vi "feux_rouge.vi"() -> ()   [LabVIEW 2018]
uses:
  F_r_var_glob.vi
panel:
  in  "stop":bool
  in  "Boolean 3":bool
  in  "Boolean 2":bool
  in  "Boolean":bool
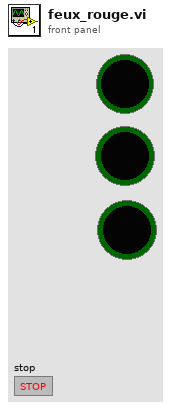
[diagram p1: front panel]
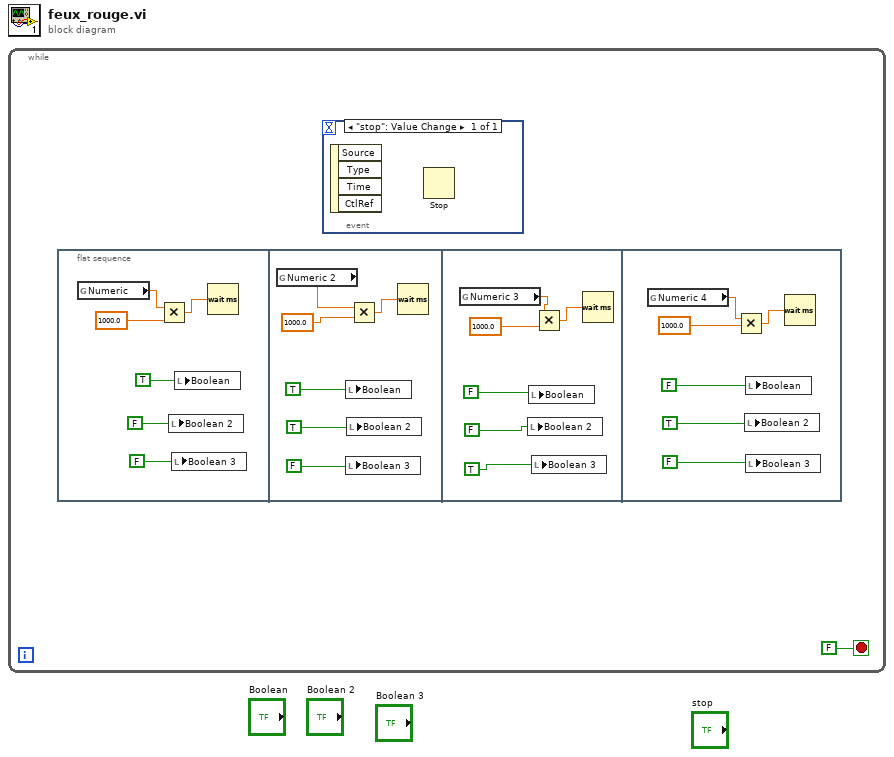
[diagram p0: block diagram]
diagram:
  n1 = while {
    stop <- FALSE stop-if-true
    n2 = flat-sequence {
      frame #0 {
        n3 = global read "F_r_var_glob.vi" "Numeric"() -> (w7:dbl)
        n4 = Multiply(x=w7, y=1000.0) -> (x*y=w5:dbl)
        n5 = local write "Boolean 2"(FALSE) -> ()
        n6 = local write "Boolean 3"(FALSE) -> ()
        n7 = local write "Boolean"(TRUE) -> ()
        n8 = Wait (ms)(milliseconds to wait=w5) -> ()  [unwired: 1 out]
      }
      frame #1 {
        n9 = global read "F_r_var_glob.vi" "Numeric 2"() -> (w11:dbl)
        n10 = local write "Boolean"(TRUE) -> ()
        n11 = local write "Boolean 3"(FALSE) -> ()
        n12 = local write "Boolean 2"(TRUE) -> ()
        n13 = Multiply(x=w11, y=1000.0) -> (x*y=w13:dbl)
        n14 = Wait (ms)(milliseconds to wait=w13) -> ()  [unwired: 1 out]
      }
      frame #2 {
        n15 = global read "F_r_var_glob.vi" "Numeric 3"() -> (w14:dbl)
        n16 = local write "Boolean 2"(FALSE) -> ()
        n17 = local write "Boolean"(FALSE) -> ()
        n18 = local write "Boolean 3"(TRUE) -> ()
        n19 = Multiply(x=w14, y=1000.0) -> (x*y=w16:dbl)
        n20 = Wait (ms)(milliseconds to wait=w16) -> ()  [unwired: 1 out]
      }
      frame #3 {
        n21 = global read "F_r_var_glob.vi" "Numeric 4"() -> (w21:dbl)
        n22 = Multiply(x=w21, y=1000.0) -> (x*y=w22:dbl)
        n23 = local write "Boolean 2"(TRUE) -> ()
        n24 = local write "Boolean"(FALSE) -> ()
        n25 = local write "Boolean 3"(FALSE) -> ()
        n26 = Wait (ms)(milliseconds to wait=w22) -> ()  [unwired: 1 out]
      }
    }
    n27 = event shown="[0] \"stop\": Value Change" {
      selector: _ -> [_]
      dyn-events: _ -> [_]
      timeout: _ -> [_]
      event "stop": Value Change {
        n28 = event-data() -> ()  [unwired: 1 in, 4 out]
        n29 = Stop() -> ()  [unwired: 1 in]
      }
    }
  }
